vi "_TangoReadAttributes.vi"(2 "error in":errorcluster, 3 "attribute names":string[](array[string]), 4 "device name":string) -> (0 "error out":errorcluster, 1 "attribute values":T3(array[cluster]))   [LabVIEW 2014, in "tango.lvlib"]
uses:
  tango.lvlib
  Common VIs/Typedefs/_AttributeQuality_t.ctl
  Common VIs/Typedefs/_AttributeDataType_t.ctl
  tango_binding.so
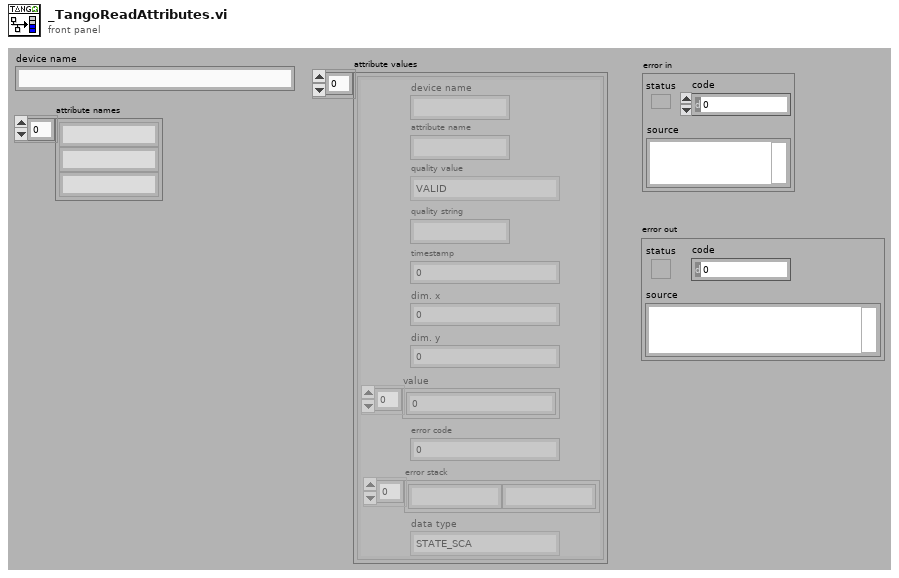
[diagram p1: front panel]
types:
  T1 = typedef "tango.lvlib/_AttributeQuality_t.ctl" = enum16{"VALID", "INVALID", "ALARM", "CHANGING", "UNKNOWN_QUALITY"}
  T2 = typedef "tango.lvlib/_AttributeDataType_t.ctl" = enum16{"STATE_SCA", "STATE_SPE", "STATE_IMG", "STRING_SCA", "STRING_SPE", "STRING_IMG", "BOOL_SCA", "BOOL_SPE", "BOOL_IMG", "UCHAR_SCA", "UCHAR_SPE", "UCHAR_IMG", "SHORT_SCA", "SHORT_SPE", "SHORT_IMG", "USHORT_SCA", "USHORT_SPE", "USHORT_IMG", "LONG_SCA", "LONG_SPE", "LONG_IMG", "ULONG_SCA", "ULONG_SPE", "ULONG_IMG", "LONG64_SCA", "LONG64_SPE", "LONG64_IMG", "ULONG64_SCA", "ULONG64_SPE", "ULONG64_IMG", "FLOAT_SCA", "FLOAT_SPE", "FLOAT_IMG", "DOUBLE_SCA", "DOUBLE_SPE", "DOUBLE_IMG", "UNKNOWN_DATA_TYPE"}
  T3 = cluster{"device name":string, "attribute name":string, "quality value":T1, "quality string":string, "timestamp":dbl, "dim. x":i32, "dim. y":i32, "value":u8[], "error code":i32, "error stack":string[], "data type":T2}[]
  T4 = cluster{"device name":string, "attribute name":string, "quality value":i16, "quality string":string, "timestamp":dbl, "dim. x":i32, "dim. y":i32, "value":u8[], "error code":i32, "error stack":string[], "data type":u16}[]
  T5 = cluster{"device name":string, "attribute name":string, "quality value":T1, "quality string":string, "timestamp":dbl, "dim. x":i32, "dim. y":i32, "value":u8[], "error code":i32, "error stack":string[], "data type":T2}
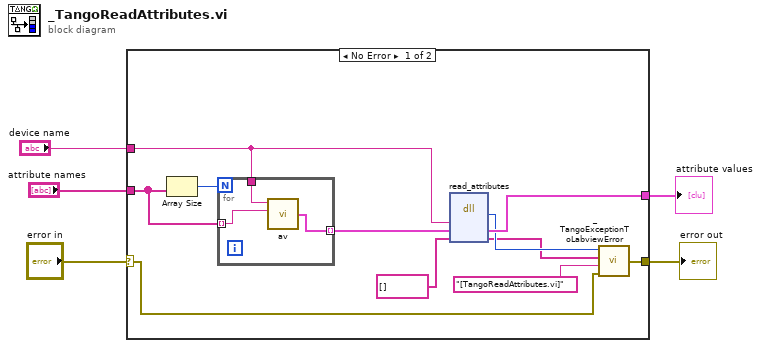
[diagram p0: block diagram]
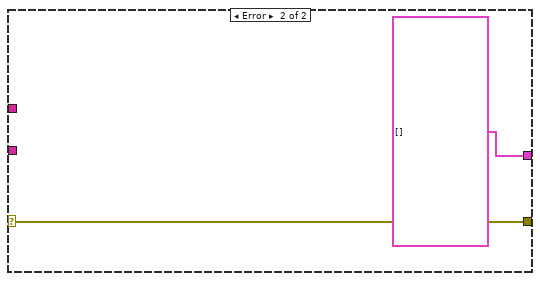
[diagram p2: hidden frame]
diagram:
  n1 = case shown="No Error" "error in" {
    selector: "error in" -> [w6 w21]
    tunnel: "attribute names" -> [w16 _]
    tunnel: "device name" -> [w15 _]
    tunnel: [w11 T4 [] ("attr_values_inout")] -> w3
    tunnel: [w7 w21] -> w1
    frame No Error {
      n2 = Array Size(array=w16) -> (size(s)=w13:i32)
      n3 = for {
        N: w13 -> [_]
        tunnel: w15 -> [w18]
        tunnel: w16 -> [w17] mode=indexing
        tunnel: [w19] -> w12 mode=indexing
        n4 = call "av.vi"("attribute name"=w17, "device name"=w18) -> ("attribute value"=w19:T5)  [unwired: 4 in]
      }
      n5 = dll-call lib="tango_binding.*" fn="read_attributes"("dev_name"=w15, "attr_values_inout"=w12, "error_stack"=string[] [] ("error stack")) -> ("return type"=w9:i32, "attr_values_inout"=w11:T3, "error_stack"=w8:string[])  [unwired: 4 in, 2 out]
      n6 = call "_TangoExceptionToLabviewError.vi"("error in"=w6, "location"="[TangoReadAttributes.vi]", "error stack"=w8, "error code"=w9) -> ("error out"=w7:errorcluster)
    }
    frame Error {
    }
  }
  "attribute values" <- w3
  "error out" <- w1
